vi "Remove Waveforms from ListBox.vi"(0 "Custom Device Ref in":T1 format="%.0x", 1 "UI Refs":T2, 5 "CD Settings in":T3 {"CD Task Dependency Ref" format="%.0x"; "CD Task Dependency" format="%.0x"}, 7 "Item Names":string[](array[string]), 9 "Value":i32[](array[numeric]), 11 "error in (no error)":errorcluster, 12 "Waveform Ref LUT":variant) -> (4 "Custom Device Ref out":T1 format="%.0x", 6 "CD Settings out":T3 {"CD Task Dependency Ref" format="%.0x"; "CD Task Dependency" format="%.0x"}, 15 "error out":errorcluster)   [LabVIEW 2015, in "Waveform-Processing-Custom-Device System Explorer.lvlib"]
uses:
  Waveform-Processing-Custom-Device System Explorer.lvlib
  Shared/Custom Device Settings.ctl
  <vilib>/NI Veristand/Custom Device API/Custom Device Item Ref.ctl
  Types/UI Refs Ctl.ctl
  <vilib>/NI Veristand/Custom Device API/Custom Device Pointer.ctl
  NationalInstruments.VeriStand.SystemStorage
  NationalInstruments.VeriStand
  <vilib>/NI Veristand/Custom Device Tools/Custom Device Utility Library/NI VeriStand - Search for Item by Name.vi
  <vilib>/NI VeriStand/Custom Device API/Custom Device API.lvlib
  <vilib>/NI VeriStand/Custom Device Tools/Custom Device Utility Library/Custom Device Utility Library.lvlib
  Shared/Waveform-Processing-Custom-Device Shared.lvlib
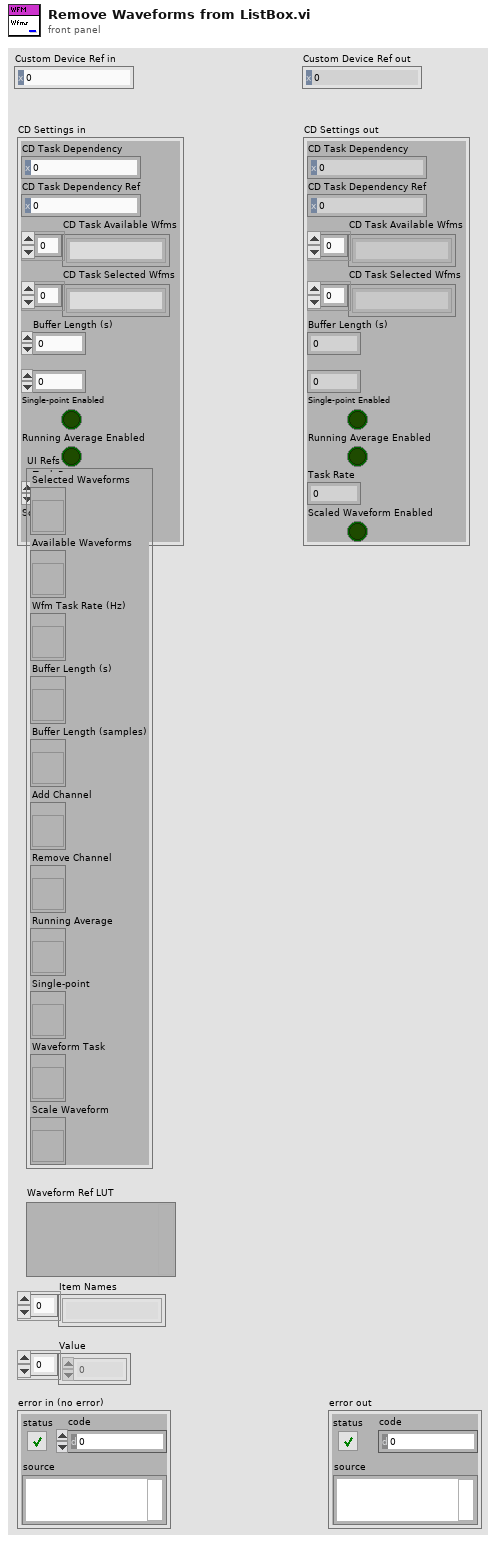
[diagram p1: front panel]
types:
  T1 = typedef "Custom Device API.lvlib/Custom Device Item Ref.ctl" = u64
  T2 = typedef "Waveform-Processing-Custom-Device Shared.lvlib/UI Refs Ctl.ctl" = cluster{"Selected Waveforms":refnum<vi>, "Available Waveforms":refnum<vi>, "Wfm Task Rate (Hz)":refnum<vi>, "Buffer Length (s)":refnum<vi>, "Buffer Length (samples)":refnum<vi>, "Add Channel":refnum<vi>, "Remove Channel":refnum<vi>, "Running Average":refnum<vi>, "Single-point":refnum<vi>, "Waveform Task":refnum<vi>, "Scale Waveform":refnum<vi>}
  T3 = typedef "Waveform-Processing-Custom-Device Shared.lvlib/Custom Device Settings.ctl" = cluster{"CD Task Dependency":T1, "CD Task Dependency Ref":T1, "CD Task Available Wfms":string[], "CD Task Selected Wfms":string[], "Buffer Length (s)":dbl, "Buffer Length (samples)":u32, "Single-point Enabled":bool, "Running Average Enabled":bool, "Task Rate":dbl, "Scaled Waveform Enabled":bool}
  T4 = typedef "Custom Device API.lvlib/Custom Device Pointer.ctl" = refnum<k24>
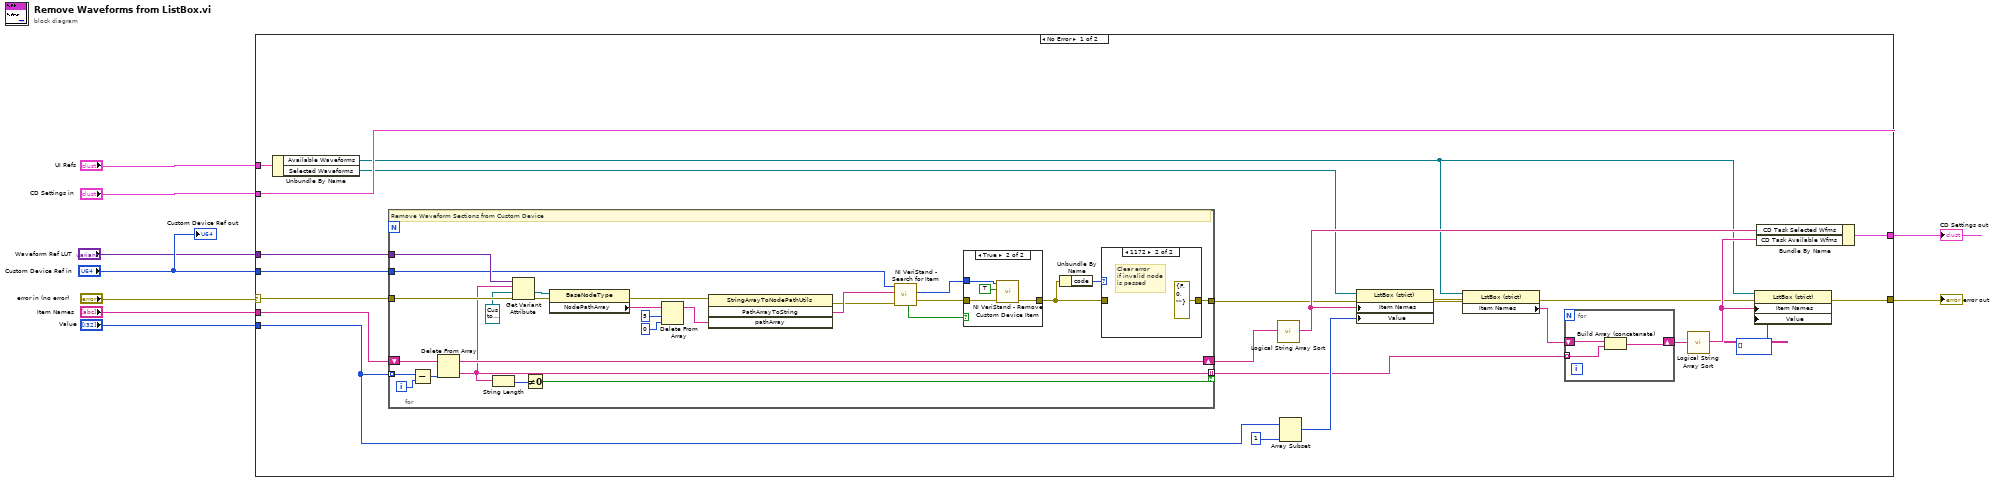
[diagram p0: block diagram]
diagram:
  n1 = case shown="No Error" "error in (no error)" {
    selector: "error in (no error)" -> [w12 w71]
    tunnel: [w24 w70] -> w9
    tunnel: "CD Settings in" -> [w23 w70]
    tunnel: [w22 w71] -> w7
    tunnel: "Item Names" -> [w18 _]
    tunnel: "Value" -> [w17 _]
    tunnel: "UI Refs" -> [w16 _]
    tunnel: "Custom Device Ref in" -> [w13 _]
    tunnel: "Waveform Ref LUT" -> [w10 _]
    frame No Error {
      n2 = Unbundle By Name(w16) -> ("Available Waveforms"=w14:refnum<vi>, "Selected Waveforms"=w15:refnum<vi>)
      n3 = for {
        tunnel: w17 -> [w59] mode=indexing
        shift-right: [w61] -> w26
        shift-left: w18 -> [w62]
        tunnel: [w50] -> w20 mode=indexing if=w57
        tunnel: w12 -> [w52]
        tunnel: w13 -> [w41]
        tunnel: [w36] -> w11
        tunnel: w10 -> [w51]
        i -> [w60]
        # "Remove Waveform Sections from Custom Device"
        n4 = Subtract(x=w59, y=w60) -> (x-y=w58:i32)
        n5 = Delete From Array(array=w62, index=w58) -> (deleted portion=w50:string, array with subset deleted=w61:string[])  [unwired: 1 in]
        n6 = String Length(string=w50) -> (length=w56:i32)
        n7 = Get Variant Attribute(Variant=w51, name=w50, default value (empty Variant)=T4 refnum ("Node Pointer"), error in=w52) -> (value=w48:T4, error out=w47:errorcluster)  [unwired: 2 out]
        n8 = Not Equal To 0?(x=w56) -> (x != 0?=w57:bool)
        n9 = property class="BaseNodeType"(reference=w48, error in=w47) -> (error out=w43:errorcluster, "NodePathArray"=w46:string[])  [unwired: 1 out]
        n10 = Delete From Array(array=w46, length=5, index=0) -> (array with subset deleted=w39:string[])  [unwired: 1 out]
        n11 = invoke class="StringArrayToNodePathUtils" method="PathArrayToString"(error in=w43, "pathArray"=w39) -> (error out=w40:errorcluster, "PathArrayToString"=w42:string)  [unwired: 2 in, 2 out]
        n12 = call-poly <vilib>:"NI VeriStand - Search for Item.vi"("error in"=w40, "Item Name"=w42, "Section Ref in"=w41) -> ("error out"=w55:errorcluster, "Item Ref"=w54:T1, "Found"=w53:bool)  [unwired: 5 in, 1 out]
        n13 = case shown="True" w53 {
          tunnel: [w65 w68] -> w37
          tunnel: w55 -> [w65 w67]
          tunnel: w54 -> [_ w66]
          frame False {
          }
          frame True {
            n14 = call <vilib>:"NI VeriStand - Remove Custom Device Item.vi"("error in (no error)"=w67, "Force Delete (F)"=TRUE, "Item Ref in"=w66) -> ("error out"=w68:errorcluster)  [unwired: 7 in, 1 out]
          }
        }
        n15 = Unbundle By Name(w37) -> ("code"=w38:i32)
        n16 = case shown="1172" w38 {
          tunnel: w37 -> [w63 _]
          tunnel: [w63 errorcluster {"status"=FALSE, "code"=0, "source"=""} ("error out")] -> w36
          frame 0, Default {
          }
          frame 1172 {
            # "Clear error\nif invalid node\nis passed"
          }
        }
      }
      n17 = call "Logical String Array Sort.vi"("Unsorted List"=w26) -> ("Sorted List"=w27:string[])  [unwired: 18 in]
      n18 = Array Subset(array=w17, length=1) -> (w31:i32[])  [unwired: 1 in]
      n19 = property on="Property Node" class="LstBox (strict)"(reference=w15, error in=w11, "Item Names"=w27, "Value"=w31) -> (error out=w19:errorcluster)  [unwired: 1 out]
      n20 = property on="Property Node" class="LstBox (strict)"(reference=w14, error in=w19) -> (error out=w21:errorcluster, "Item Names"=w25:string[])  [unwired: 1 out]
      n21 = for {
        tunnel: w20 -> [w34] mode=indexing
        shift-right: [w33] -> w28
        shift-left: w25 -> [w35]
        n22 = Build Array (concatenate)(w35, w34) -> (w33:string[])
      }
      n23 = call "Logical String Array Sort.vi"("Unsorted List"=w28) -> ("Sorted List"=w29:string[])  [unwired: 18 in]
      n24 = property on="Property Node" class="LstBox (strict)"(reference=w14, error in=w21, "Item Names"=w29, "Value"=i32[] [] ("Waveforms to Process")) -> (error out=w22:errorcluster)  [unwired: 1 out]
      n25 = Bundle By Name(cluster=w23, "CD Task Selected Wfms"=w27, "CD Task Available Wfms"=w29) -> (w24:T3)
    }
    frame Error {
    }
  }
  "CD Settings out" <- w9
  "error out" <- w7
  "Custom Device Ref out" <- "Custom Device Ref in"
